vi "PM5000_VIF_Power.vi"(8 "error in":errorcluster, 11 "Network Path":string="172.22.26.202") -> (0 "error out":errorcluster, 2 "VIF_cluster":T1, 3 "Network Path out":string="192.168.169.1")   [LabVIEW 2018]
doc: "Lee la tabla de memoria RealTime_VIF_Power del equipo PowerMonitor 5000, ademas filtra y ordena las variables de interez de la tabla de memoria.\n\nLee las siguientes variables de la tabla RealTime_VIF_Power:\n\n*V1_V2_Volts\n*V2_V3_Volts\n*V3_V1_Volts\n*I1_Amps\n*I2_Amps\n*I3_Amps\n*Frequency_Hz\n*Total_kW\n*Total_kVAR\n*Total_kVA\n*Total_True_PF\n*Total_Disp_PF"
uses:
  Controls/VIF_cluster.ctl
  <vilib>/ethernetip/ethernetip.llb/EthernetIP SLC500 Read Float.vi
  <vilib>/ethernetip/ethernetip.lvlib
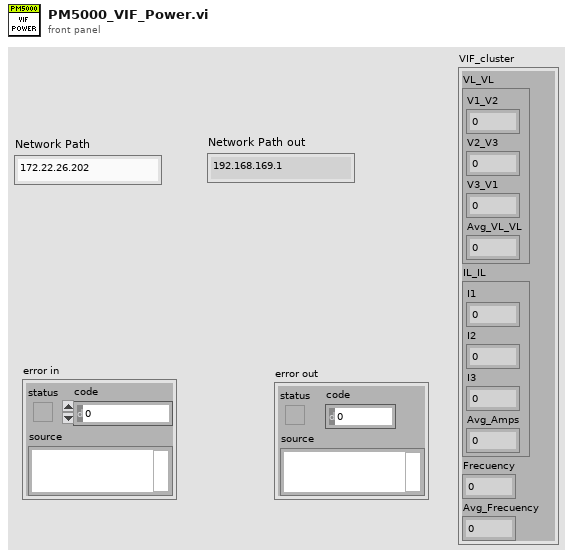
[diagram p1: front panel]
types:
  T1 = typedef "VIF_cluster.ctl" = cluster{"VL_VL":cluster{"V1_V2":sgl, "V2_V3":sgl, "V3_V1":sgl, "Avg_VL_VL":sgl}, "IL_IL":cluster{"I1":sgl, "I2":sgl, "I3":sgl, "Avg_Amps":sgl}, "Frecuency":sgl, "Avg_Frecuency":sgl}
  T2 = cluster{"I1 (A)":sgl, "I2 (A)":sgl, "I3 (A)":sgl, "Avg_Amps":sgl}
  T3 = cluster{"V1_V2 (V)":sgl, "V2_V3 (V)":sgl, "V3_V1 (V)":sgl, "Avg_VL_VL":sgl}
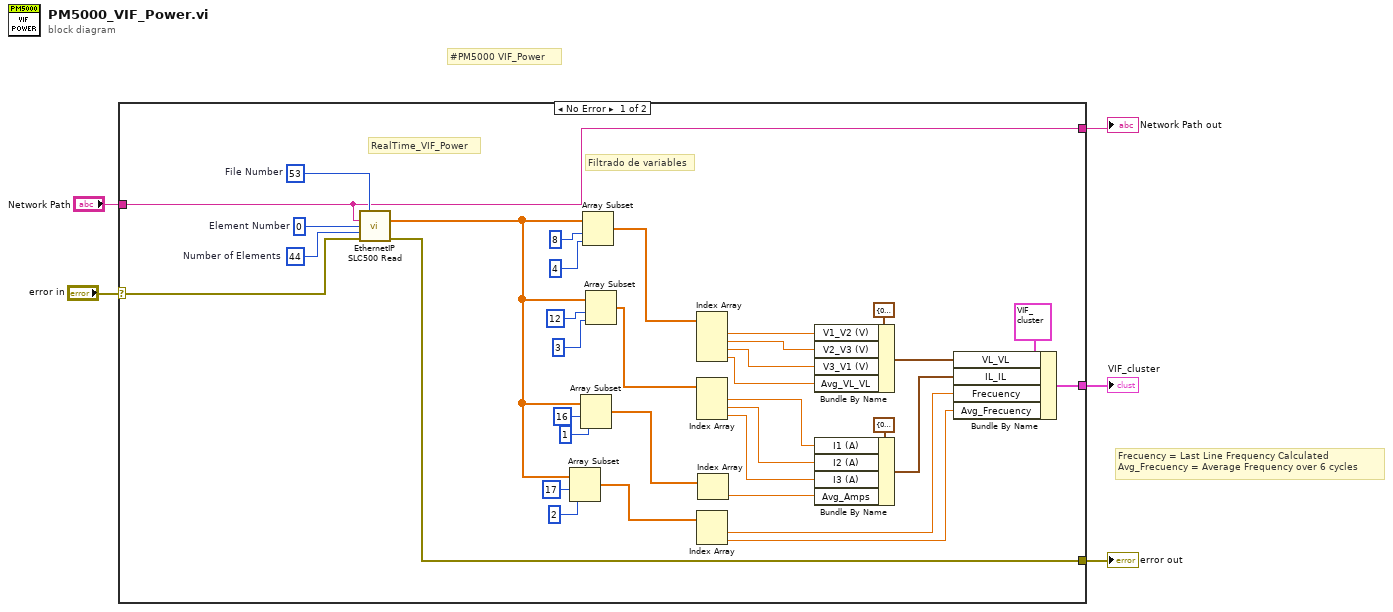
[diagram p0: block diagram]
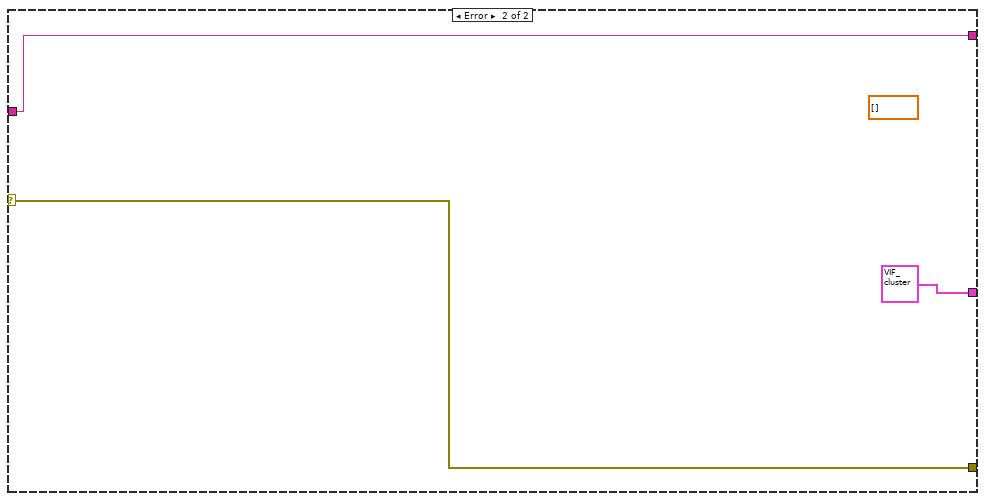
[diagram p2: hidden frame]
diagram:
  # "Frecuency = Last Line Frequency Calculated\nAvg_Frecuency = Average Frequency over 6 cycles"
  # "#PM5000 VIF_Power"
  n1 = case shown="No Error" "error in" {
    selector: "error in" -> [w32 w43]
    tunnel: [w37 w43] -> w5
    tunnel: [w26 T1 {"VL_VL"={"V1_V2"=0.0, "V2_V3"=0.0, "V3_V1"=0.0, "Avg_VL_VL"=0.0}, "IL_IL"={"I1"=0.0, "I2"=0.0, "I3"=0.0, "Avg_Amps"=0.0}, "Frecuency"=0.0, "Avg_Frecuency"=0.0} ("VIF_cluster")] -> w3
    tunnel: [w19 w41] -> w2
    tunnel: "Network Path" -> [w19 w41]
    frame No Error {
      w38 = u32 44  # Number of Elements
      w40 = u16 53  # File Number
      w39 = u16 0  # Element Number
      # "Filtrado de variables"
      # "RealTime_VIF_Power"
      n2 = call-poly <vilib>:"EthernetIP SLC500 Read.vi"("File Number"=w40, "Network Path"=w19, "Element Number"=w39, "Number of Elements"=w38, "error in"=w32) -> ("Data"=w13:sgl[], "error out"=w37:errorcluster)  [unwired: 8 in, 1 out]
      n3 = Array Subset(array=w13, index=17, length=2 ("index")) -> (w10:sgl[])
      n4 = Array Subset(array=w13, index=16, length=1) -> (w15:sgl[])
      n5 = Array Subset(array=w13, index=8, length=4) -> (w31:sgl[])
      n6 = Array Subset(array=w13, index=12, length=3) -> (w30:sgl[])
      n7 = Index Array(array=w31) -> (element #1=w25:sgl, element #2=w24:sgl, element #3=w23:sgl, element #4=w18:sgl)  [unwired: 4 in]
      n8 = Index Array(array=w30) -> (element #1=w22:sgl, element #2=w21:sgl, element #3=w20:sgl)  [unwired: 3 in]
      n9 = Index Array(array=w10) -> (element #1=w7:sgl, element #2=w6:sgl)  [unwired: 2 in]
      n10 = Index Array(array=w15) -> (element=w14:sgl)  [unwired: 1 in]
      n11 = Bundle By Name(cluster=T3 {"V1_V2 (V)"=0.0, "V2_V3 (V)"=0.0, "V3_V1 (V)"=0.0, "Avg_VL_VL"=0.0} ("VL_VL"), "V1_V2 (V)"=w25, "V2_V3 (V)"=w24, "V3_V1 (V)"=w23, "Avg_VL_VL"=w18) -> (w9:T3)
      n12 = Bundle By Name(cluster=T2 {"I1 (A)"=0.0, "I2 (A)"=0.0, "I3 (A)"=0.0, "Avg_Amps"=0.0} ("IL_IL"), "I1 (A)"=w22, "I2 (A)"=w21, "I3 (A)"=w20, "Avg_Amps"=w14) -> (w8:T2)
      n13 = Bundle By Name(cluster=T1 {"VL_VL"={"V1_V2"=0.0, "V2_V3"=0.0, "V3_V1"=0.0, "Avg_VL_VL"=0.0}, "IL_IL"={"I1"=0.0, "I2"=0.0, "I3"=0.0, "Avg_Amps"=0.0}, "Frecuency"=0.0, "Avg_Frecuency"=0.0} ("VIF_cluster"), "VL_VL"=w9, "IL_IL"=w8, "Frecuency"=w7, "Avg_Frecuency"=w6) -> (w26:T1)
    }
    frame Error {
      (unwired) sgl[] []
    }
  }
  "error out" <- w5
  "VIF_cluster" <- w3
  "Network Path out" <- w2
